vi "Disabled.vi"(7 "Robot Mode":T2, 10 "Match Info":T1={"Autonomous Elapsed Seconds"=0.0, "TeleOp Elapsed Seconds"=0.0, "Disabled Elapsed Seconds"=0.0, "Visited Autonomous"=FALSE, "Visited TeleOp"=FALSE, "Visited Disabled"=FALSE, "Autonomous Settings"={"Autonomous Style"=enum."Independent", "VI Refnum"=refnum}}, 11 "Call Context":T3) -> ()   [LabVIEW 2016]
doc: "This VI is called each time a disabled packet is received from the DS. It is often used to prepare for the next robot mode, to calibrate sensors, etc."
uses:
  <vilib>/Rock Robotics/WPI/DriverStation/WPI_DriverStationDerivedRobotMode.ctl
  <vilib>/Rock Robotics/WPI/DriverStation/WPI_DriverStationRobotMode2.ctl
  <vilib>/Rock Robotics/WPI/DriverStation/WPI_DriverStationMatch Info.ctl
  Robot Global Data.vi
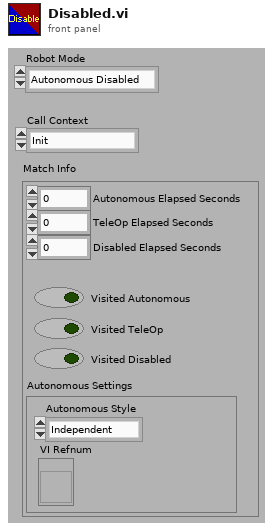
[diagram p1: front panel]
types:
  T1 = typedef "WPI_DriverStationMatch Info.ctl" = cluster{"Autonomous Elapsed Seconds":dbl, "TeleOp Elapsed Seconds":dbl, "Disabled Elapsed Seconds":dbl, "Visited Autonomous":bool, "Visited TeleOp":bool, "Visited Disabled":bool, "Autonomous Settings":cluster{"Autonomous Style":enum16{"Iterative", "Independent"}, "VI Refnum":refnum<vi>}}
  T2 = typedef "WPI_DriverStationRobotMode2.ctl" = enum16{"Autonomous Disabled", "Autonomous Enabled", "Teleop Disabled", "Teleop Enabled", "Disconnected", "Finish", "Test Disabled", "Test Enabled", "Emergency Stopped"}
  T3 = typedef "WPI_DriverStationDerivedRobotMode.ctl" = enum16{"Init", "Execute", "Stop"}
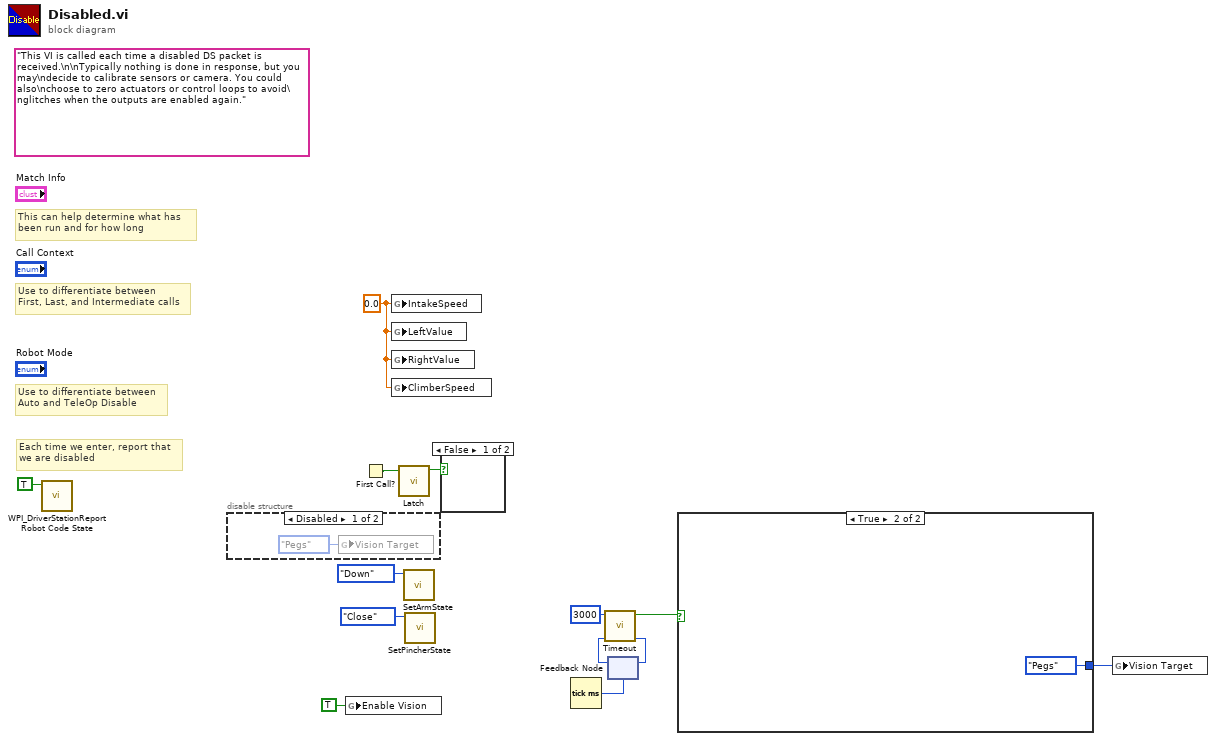
[diagram p0: block diagram]
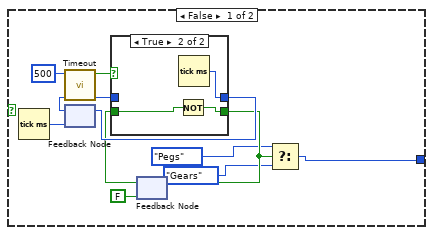
[diagram p2: hidden frame]
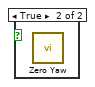
[diagram p5: hidden frame]
diagram:
  w12 = 0.0 ("ClimberSpeed")
  (unwired) "This VI is called each time a disabled DS packet is received.\n\nTypically nothing is done in response, but you may\ndecide to calibrate sensors or camera. You could also\nchoose to zero actuators or control loops to avoid\nglitches when the outputs are enabled again."
  # "Each time we enter, report that\nwe are disabled"
  # "Use to differentiate between\nFirst, Last, and Intermediate calls"
  # "This can help determine what has\nbeen run and for how long"
  # "Use to differentiate between\nAuto and TeleOp Disable"
  n1 = call <vilib>:"WPI_DriverStationReport Robot Code State.vi"("Disabled"=TRUE ("Autonomous")) -> ()  [unwired: 10 in, 1 out]
  n2 = disable-structure shown="Disabled" {
    frame Disabled {
      n3 = global write "Robot Global Data.vi" "Vision Target"(enum16{"Pegs", "Gears"}."Pegs" ("Vision Target")) -> ()
    }
    frame Enabled {
    }
  }
  n4 = global write "Robot Global Data.vi" "Enable Vision"(TRUE ("Enable Vision")) -> ()
  n5 = First Call?() -> (First Call?: T/F=w1:bool)
  n6 = global write "Robot Global Data.vi" "IntakeSpeed"(w12) -> ()
  n7 = global write "Robot Global Data.vi" "LeftValue"(w12) -> ()
  n8 = global write "Robot Global Data.vi" "RightValue"(w12) -> ()
  n9 = global write "Robot Global Data.vi" "ClimberSpeed"(w12) -> ()
  n10 = call "Latch.vi"("Input"=w1) -> ("Output"=w11:bool)  [unwired: 10 in]
  n11 = call "SetArmState.vi"("ArmState"=enum16{"Up", "Down"}."Down") -> ()  [unwired: 10 in, 1 out]
  n12 = call "SetPincherState.vi"("PincherState"=enum16{"Open", "Close"}."Close") -> ()  [unwired: 10 in, 1 out]
  n13 = case shown="False" w11 {
    frame False {
    }
    frame True {
      n14 = call <vilib>:"Zero Yaw.vi"() -> ()  [unwired: 12 in]
    }
  }
  n15 = Tick Count (ms)() -> (millisecond timer value=w2:u32)
  n16 = feedback #1(w2) -> (w3:u32)
  n17 = call "Timeout.vi"("Start Time In"=w3, "Time Limit"=u32 3000) -> ("Start Time Out"=w4:u32, "Timeout"=w6:bool)  [unwired: 8 in]
  n18 = feedback-in #1(w4) -> ()
  n19 = case shown="True" w6 {
    tunnel: [w15 enum16{"Pegs", "Gears"}."Pegs" ("Vision Target")] -> w5
    frame False {
      n20 = Tick Count (ms)() -> (millisecond timer value=w24:u32)
      n21 = feedback #2(w24) -> (w22:u32)
      n22 = call "Timeout.vi"("Start Time In"=w22, "Time Limit"=u32 500) -> ("Start Time Out"=w25:u32, "Timeout"=w26:bool)  [unwired: 8 in]
      n23 = feedback #3(FALSE) -> (w20:bool)
      n24 = case shown="True" w26 {
        tunnel: w20 -> [w28 w31]
        tunnel: [w28 w30] -> w21
        tunnel: w25 -> [w27 _]
        tunnel: [w27 w29] -> w23
        frame False {
        }
        frame True {
          n25 = Not(x=w31) -> (.not. x?=w30:bool)
          n26 = Tick Count (ms)() -> (millisecond timer value=w29:u32)
        }
      }
      n27 = feedback-in #2(w23) -> ()
      n28 = feedback-in #3(w21) -> ()
      n29 = Select(t=enum16{"Pegs", "Gears"}."Pegs" ("Vision Target"), s=w21, f=enum16{"Pegs", "Gears"}."Gears" ("Vision Target")) -> (s? t:f=w15:enum16{"Pegs", "Gears"})
    }
    frame True {
    }
  }
  n30 = global write "Robot Global Data.vi" "Vision Target"(w5) -> ()
